vi "EncoderVelocity (1).vi"(8 "Time @(n-1)":dbl, 9 "Time @n":dbl, 10 "Encoder Distance (mm) @n-1":dbl, 11 "Encoder Distance (mm) @n":dbl) -> (3 "Encoder Speed (mm/s)":dbl)   [LabVIEW 2013]
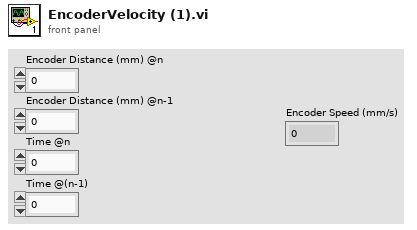
[diagram p1: front panel]
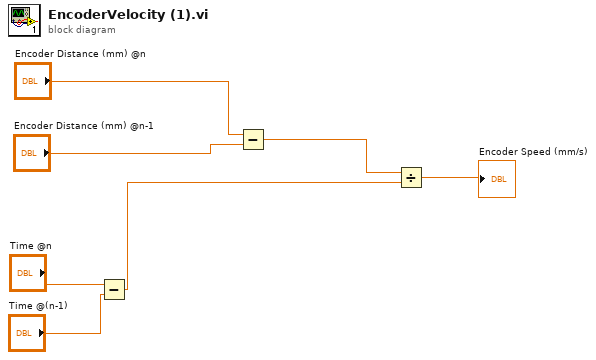
[diagram p0: block diagram]
diagram:
  n1 = Subtract(x="Time @n", y="Time @(n-1)") -> (x-y=w3:dbl)
  n2 = Subtract(x="Encoder Distance (mm) @n", y="Encoder Distance (mm) @n-1") -> (x-y=w5:dbl)
  n3 = Divide(x=w5, y=w3) -> (x/y=→"Encoder Speed (mm/s)":dbl)
